vi "Read RFmx VNA Session.vi"(8 "error in (no error)":errorcluster, 11 "Vector Path in":refnum<class "Vector Path.lvclass">) -> (0 "error out":errorcluster, 2 "RFmx VNA Session":refnum<k21>, 3 "Vector Path out":refnum<class "Vector Path.lvclass">)   [LabVIEW 2023, in "RFFixtureCharact.Public.lvlib" / "Vector Path.lvclass"]
uses:
  Vector Path.lvclass
  Vector Path.lvclass/Vector Path.ctl
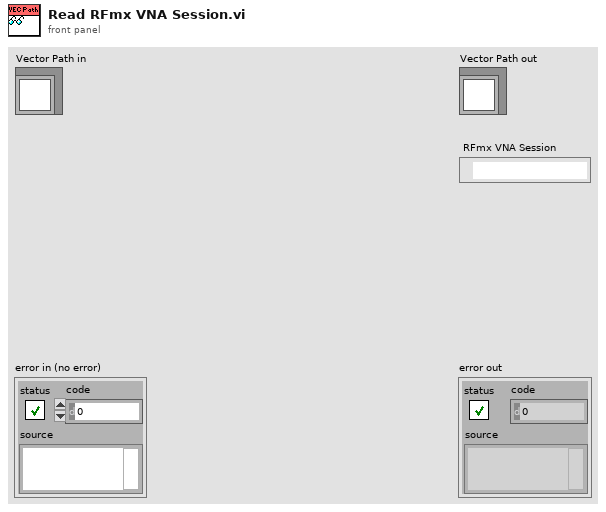
[diagram p1: front panel]
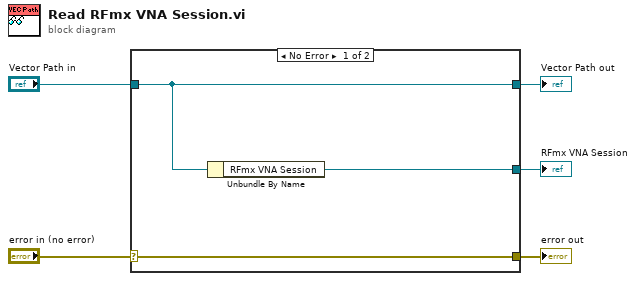
[diagram p0: block diagram]
diagram:
  n1 = case shown="No Error" "error in (no error)" {
    selector: "error in (no error)" -> [w8 w9]
    tunnel: [w8 w9] -> w4
    tunnel: [w7 w10] -> w2
    tunnel: "Vector Path in" -> [w7 w10]
    tunnel: [w6 _] -> w1
    frame No Error {
      n2 = Unbundle By Name(w7) -> ("RFmx VNA Session"=w6:refnum<k21>)
    }
    frame Error {
    }
  }
  "error out" <- w4
  "Vector Path out" <- w2
  "RFmx VNA Session" <- w1
